vi "Testing.vi"() -> ()   [LabVIEW 2014]
panel:
  out "x-y*floor(x/y)":dbl
  in  "x":dbl
  in  "y":dbl
  out "floor(x/y)":u8
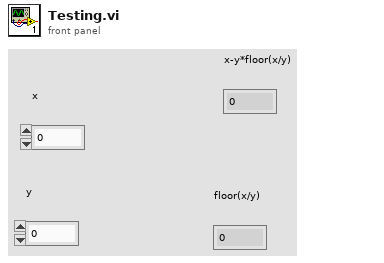
[diagram p1: front panel]
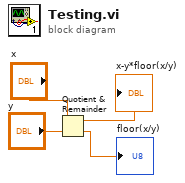
[diagram p0: block diagram]
diagram:
  n1 = Quotient & Remainder(x="x", y="y") -> (x-y*floor(x/y)=→"x-y*floor(x/y)":dbl, floor(x/y)=→"floor(x/y)":dbl)
